vi "close.vi"(8 "error in (no error)":errorcluster caption="错误输入（无错误）", 11 "access 输入":refnum<class "access.lvclass">) -> (0 "error out":errorcluster caption="错误输出", 3 "access 输出":refnum<class "access.lvclass">)   [LabVIEW 2016, in "潮位站数据传输.lvlib" / "access.lvclass"]
uses:
  access.lvclass
  <vilib>/addons/database/NI_Database_API.lvlib
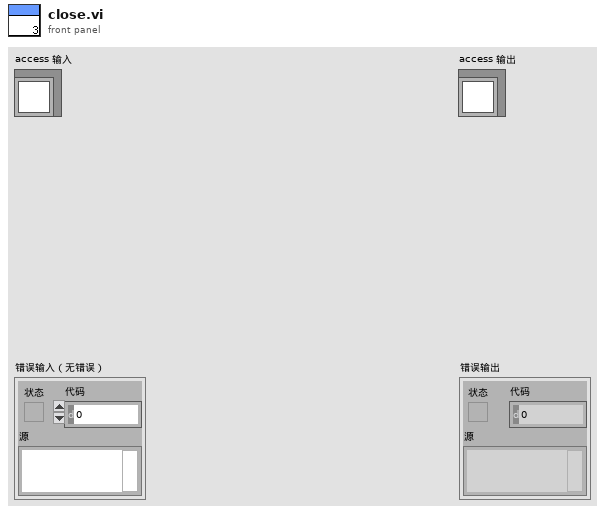
[diagram p1: front panel]
types:
  T1 = typedef "NI_Database_API.lvlib/Conn ObjectReference.ctl" = refnum<k1>
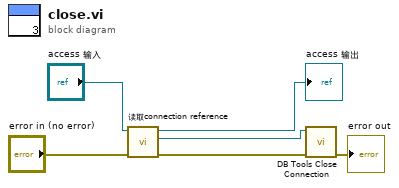
[diagram p0: block diagram]
diagram:
  n1 = call-dynamic "读取connection reference.vi"("error in (no error)"="error in (no error)", "database输入"="access 输入") -> ("error out"=w1:errorcluster, "reference"=w2:T1, "database输出"=→"access 输出":refnum<class "access.lvclass">)  [unwired: 7 in]
  n2 = call <vilib>:"DB Tools Close Connection.vi"("error in (no error)"=w1, "connection reference"=w2) -> ("error out"=→"error out":errorcluster)  [unwired: 5 in]
